vi "AWS Credentials.vi"() -> ()   [LabVIEW 2014, in "FRCts20_Backend_Engine.lvlib"]
uses:
  FRCts20_Backend_Engine.lvlib
  <vilib>/National Instruments/NI Amazon Web Services (AWS) Toolkit for LabVIEW/S3/vi source/Typedefs/AMZ_S3_AWS Credentials.ctl
  <vilib>/National Instruments/NI Amazon Web Services (AWS) Toolkit for LabVIEW/S3/vi source/LV Interface for Amazon S3.lvlib
panel:
  in  "Bucket":string="parkway_avatars"
  in  "AWS Credentials in":T1={"Access Key"="AKIAI4UOFGXQQ2XM3KTQ", "Secret Key"="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"}
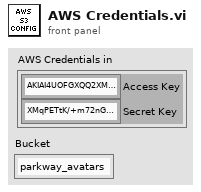
[diagram p1: front panel]
types:
  T1 = typedef "LV Interface for Amazon S3.lvlib/AMZ_S3_AWS Credentials.ctl" = cluster{"Access Key":string, "Secret Key":string}
diagram:
